vi "execute.vi"(8 "error in (no error)":errorcluster, 10 "ComponentData.lvclass":refnum<class "ComponentData.lvclass">, 11 "ComponentState in":refnum<class "ComponentState.lvclass">) -> (0 "error out":errorcluster, 2 "ComponentData.lvclass 2":refnum<class "ComponentData.lvclass">, 3 "ComponentState out":refnum<class "ComponentState.lvclass">)   [LabVIEW 2013, in "ComponentData.lvlib" / "ComponentState.lvclass"]
uses:
  <userlib>/Common/Component/common_application/RT/ComponentData/ComponentState/ComponentState/ComponentState.lvclass
  <userlib>/Common/Component/common_application/RT/ComponentData/ComponentData/ComponentData.lvclass
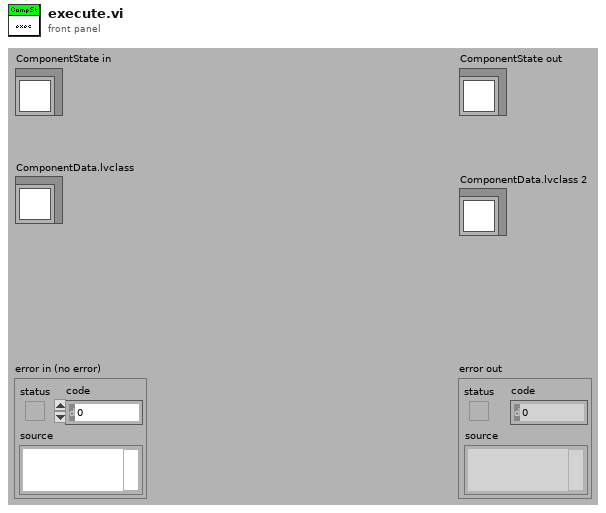
[diagram p1: front panel]
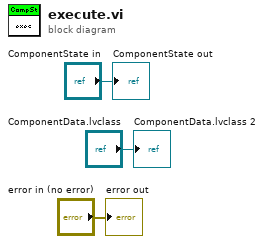
[diagram p0: block diagram]
diagram:
  "error out" <- "error in (no error)"
  "ComponentState out" <- "ComponentState in"
  "ComponentData.lvclass 2" <- "ComponentData.lvclass"
